vi "Initialize Instrument.vi"(8 "error in (no error)":errorcluster, 10 "Instrument Address":string, 11 "Instrument in":refnum<class "Instrument.lvclass">) -> (0 "error out":errorcluster, 3 "Instrument out":refnum<class "Instrument.lvclass">)   [LabVIEW 2017, in "Instrument.lvlib" / "Instrument.lvclass"]
doc: "Connects the PC to the instrument located at \"Instrument Address\" and initializes it to a known state. Instrument Address can be any string, or string-compatible physical device address [i.e. DAQmx address, VISA address,"
uses:
  Instrument.lvclass
  Instrument.lvclass/Instrument.ctl
  Properties/Instrument Properties.lvclass/Instrument Properties.ctl
  Properties/Instrument Properties.lvclass
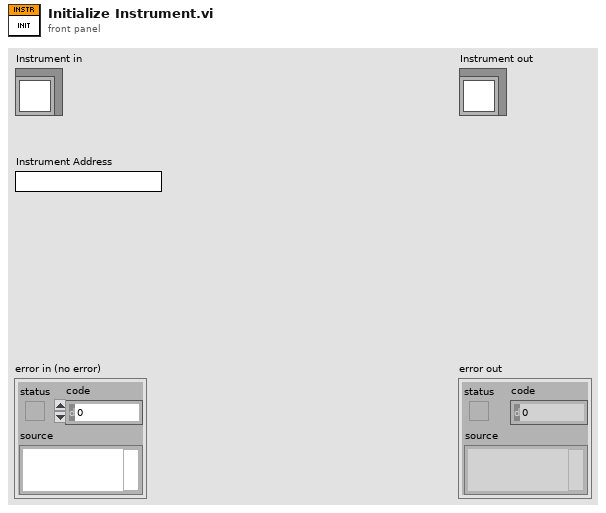
[diagram p1: front panel]
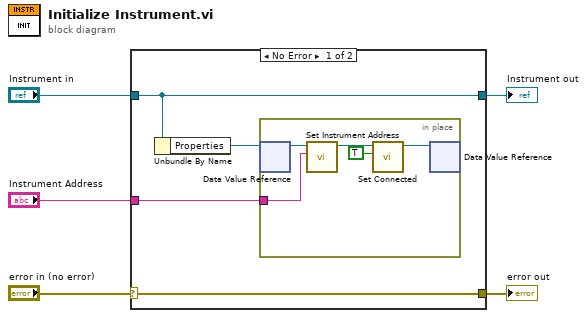
[diagram p0: block diagram]
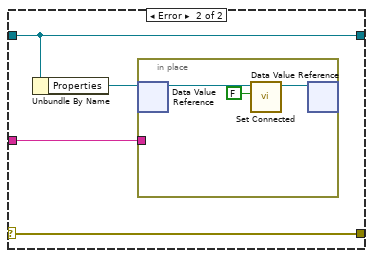
[diagram p2: hidden frame]
diagram:
  n1 = case shown="No Error" "error in (no error)" {
    selector: "error in (no error)" -> [w9 w18]
    tunnel: [w9 w18] -> w4
    tunnel: [w8 w17] -> w2
    tunnel: "Instrument in" -> [w8 w17]
    tunnel: "Instrument Address" -> [w6 w15]
    frame No Error {
      n2 = Unbundle By Name(w8) -> ("Properties"=w7:refnum<data-value>)
      n3 = in-place {
        in-place-border: w6 -> [w13]
        n4 = in-place-dvr #1(w7) -> (w14:refnum<class "Instrument Properties.lvclass">)  [unwired: 1 out]
        n5 = call-dynamic "Set Instrument Address.vi"("Instrument Address"=w13, "Instrument Properties in"=w14) -> ("Instrument Properties out"=w12:refnum<class "Instrument Properties.lvclass">)  [unwired: 8 in, 1 out]
        n6 = call "Set Connected.vi"("Connected"=TRUE, "Instrument Properties in"=w12) -> ("Instrument Properties out"=w11:refnum<class "Instrument Properties.lvclass">)  [unwired: 8 in, 1 out]
        n7 = in-place-dvr #1(w11) -> ()  [unwired: 2 out]
      }
    }
    frame Error {
      n8 = Unbundle By Name(w17) -> ("Properties"=w16:refnum<data-value>)
      n9 = in-place {
        in-place-border: w15 -> [_]
        n10 = in-place-dvr #2(w16) -> (w19:refnum<class "Instrument Properties.lvclass">)  [unwired: 1 out]
        n11 = call "Set Connected.vi"("Connected"=FALSE, "Instrument Properties in"=w19) -> ("Instrument Properties out"=w21:refnum<class "Instrument Properties.lvclass">)  [unwired: 8 in, 1 out]
        n12 = in-place-dvr #2(w21) -> ()  [unwired: 2 out]
      }
    }
  }
  "error out" <- w4
  "Instrument out" <- w2
